vi "pump rpm (mL per min).vi"(0 "Pump":T1 {"flow rate" format="%.2f"}) -> (2 "pump speed":dbl[unit] format="%.2f", 3 "pump speed (rpm)":dbl format="%.2f", 4 "tube diameter":dbl[unit] format="%.2f", 5 "in range":bool)   [LabVIEW 2012]
panel:
  in  "diameter":dbl[unit][](array[numeric])=[0.00079375, 0.0015875, 0.003175, 0.004762499999999999, 0.00635, 0.0079375] format="%.5f"
  in  "pumpflow":dbl[unit][](array[numeric])=[9.549296547316535e-09, 3.342253804929783e-08, 1.2732395447351617e-07, 2.705634032562094e-07, 4.4563384065730255e-07, 6.04788783748884e-07] format="%.3f"
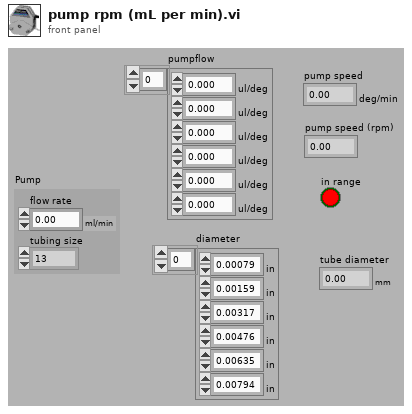
[diagram p1: front panel]
types:
  T1 = cluster{"tubing size":enum16{"13", "14", "16", "25", "17", "18"}, "flow rate":dbl[unit]}
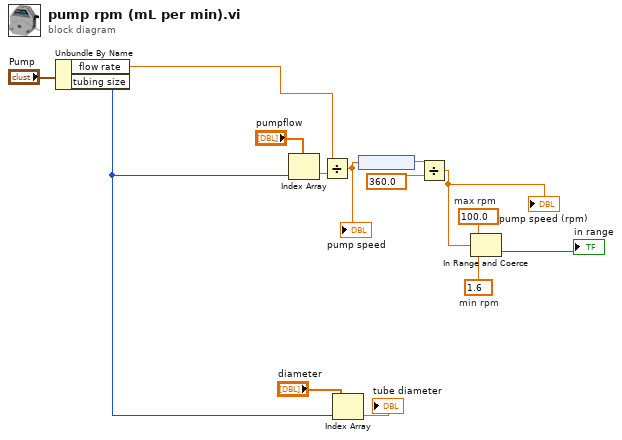
[diagram p0: block diagram]
diagram:
  w6 = 1.6  # min rpm
  w7 = 100.0  # max rpm
  n1 = Unbundle By Name("Pump") -> ("flow rate"=w1:dbl[unit], "tubing size"=w2:enum16{"13", "14", "16", "25", "17", "18"})
  n2 = Index Array(array="pumpflow", index=w2) -> (element=w13:dbl[unit])
  n3 = Divide(x=w1, y=w13) -> (x/y=w12:dbl[unit])
  "pump speed" <- w12
  n4 = Index Array(array="diameter", index=w2) -> (element=→"tube diameter":dbl[unit])
  n5 = node(w12) -> (w11:dbl)
  n6 = Divide(x=w11, y=360.0) -> (x/y=w4:dbl)
  "pump speed (rpm)" <- w4
  n7 = In Range and Coerce(upper limit=w7, x=w4, lower limit=w6) -> (In Range?=→"in range":bool)  [unwired: 1 out]
